vi "Set_Dynamic_Data_Cluster.vi"() -> ()   [LabVIEW 2023]
panel:
  in  "Numeric 32":dbl
  in  "Numeric 31":dbl
  in  "Numeric 30":dbl
  in  "Numeric 29":dbl
  in  "Numeric 28":dbl
  in  "Numeric 27":dbl
  in  "Numeric 26":dbl
  in  "Numeric 25":dbl
  in  "Numeric 24":dbl
  in  "Numeric 23":dbl
  in  "Numeric 22":dbl
  in  "Numeric 21":dbl
  in  "Numeric 20":dbl
  in  "Numeric 19":dbl
  in  "Numeric 18":dbl
  in  "Numeric 17":dbl
  in  "Numeric 16":dbl
  in  "Numeric 15":dbl
  in  "Numeric 14":dbl
  in  "Numeric 13":dbl
  in  "Numeric 12":dbl
  in  "Numeric 11":dbl
  in  "Numeric 10":dbl
  in  "Numeric 9":dbl format="%#_13g"
  in  "Numeric 8":dbl
  in  "Numeric 7":dbl
  in  "Numeric 6":dbl format="%#_13g"
  in  "Numeric 5":dbl
  in  "Numeric 4":dbl
  in  "Numeric 3":dbl
  in  "Numeric 2":dbl format="%#_13g"
  in  "Numeric":dbl
  in  "OK Button":bool
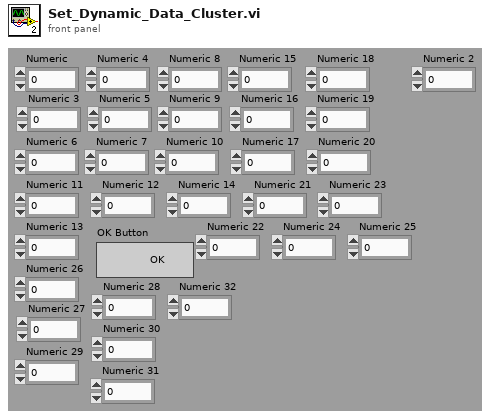
[diagram p1: front panel]
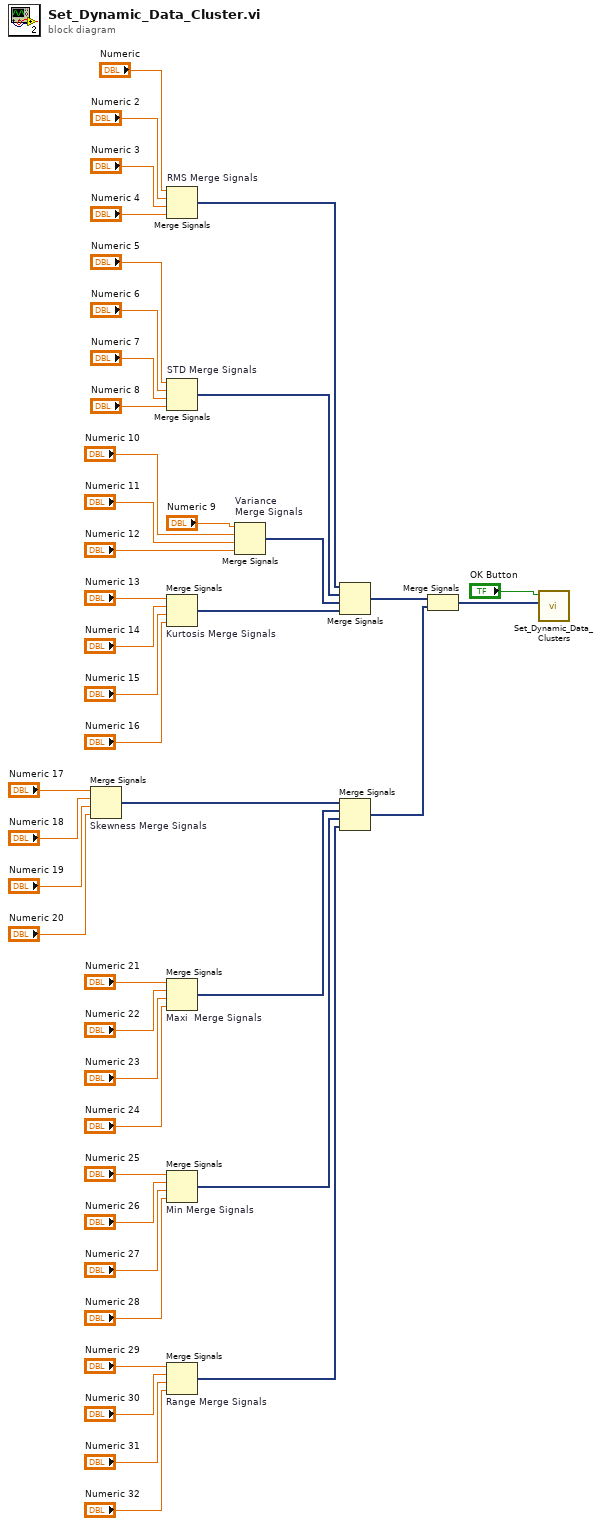
[diagram p0: block diagram]
diagram:
  n1 = Merge Signals "Skewness Merge Signals"("Numeric 17", "Numeric 18", "Numeric 19", "Numeric 20") -> (w37:dynamicdata)
  n2 = Merge Signals "RMS Merge Signals"("Numeric", "Numeric 2", "Numeric 3", "Numeric 4") -> (w41:dynamicdata)
  n3 = Merge Signals "STD Merge Signals"("Numeric 5", "Numeric 6", "Numeric 7", "Numeric 8") -> (w40:dynamicdata)
  n4 = Merge Signals "Kurtosis Merge Signals"("Numeric 13", "Numeric 14", "Numeric 15", "Numeric 16") -> (w38:dynamicdata)
  n5 = Merge Signals "Maxi  Merge Signals"("Numeric 21", "Numeric 22", "Numeric 23", "Numeric 24") -> (w36:dynamicdata)
  n6 = Merge Signals "Min Merge Signals"("Numeric 25", "Numeric 26", "Numeric 27", "Numeric 28") -> (w35:dynamicdata)
  n7 = Merge Signals "Range Merge Signals"("Numeric 29", "Numeric 30", "Numeric 31", "Numeric 32") -> (w34:dynamicdata)
  n8 = Merge Signals "Variance \nMerge Signals"("Numeric 9", "Numeric 10", "Numeric 11", "Numeric 12") -> (w39:dynamicdata)
  n9 = Merge Signals "Merge Signals"(w41, w40, w39, w38) -> (w42:dynamicdata)
  n10 = Merge Signals "Merge Signals"(w37, w36, w35, w34) -> (w33:dynamicdata)
  n11 = Merge Signals(w42, w33) -> (w43:dynamicdata)
  n12 = call "Set_Dynamic_Data_Clusters.vi"("Dynamic Data"=w43, "OK Button"="OK Button") -> ()  [unwired: 10 in]
